vi "REWORK_add_values_to_operations.vi"(7 "REPORT_all_info":T1, 10 "operation_statuses":T3[](array[typedef]), 11 "operations":string[][](array[string])) -> (2 "record_statuses":T3[](array[typedef]), 3 "ItemNames":string[][](array[string]))   [LabVIEW 2019]
uses:
  REWORK_gear_statuses.ctl
  REWORK_all_info.ctl
  MAIN/REWORK_header_data_display.ctl
  REWORK_references.ctl
  <userlib>/_OpenG.lib/array/array.llb/Reverse 2D Array (String)__ogtk.vi
  <userlib>/_OpenG.lib/array/array.llb/Filter 1D Array with Scalar (String)__ogtk.vi
  _misc/AULocalize/SubVIs/Get Localized Phrase Compact Interface 1D.vi
  _misc/AULocalize/SubVIs/Get Localized Phrase Compact Interface 2D.vi
panel:
  # "GEAR INFO SUMMARY"
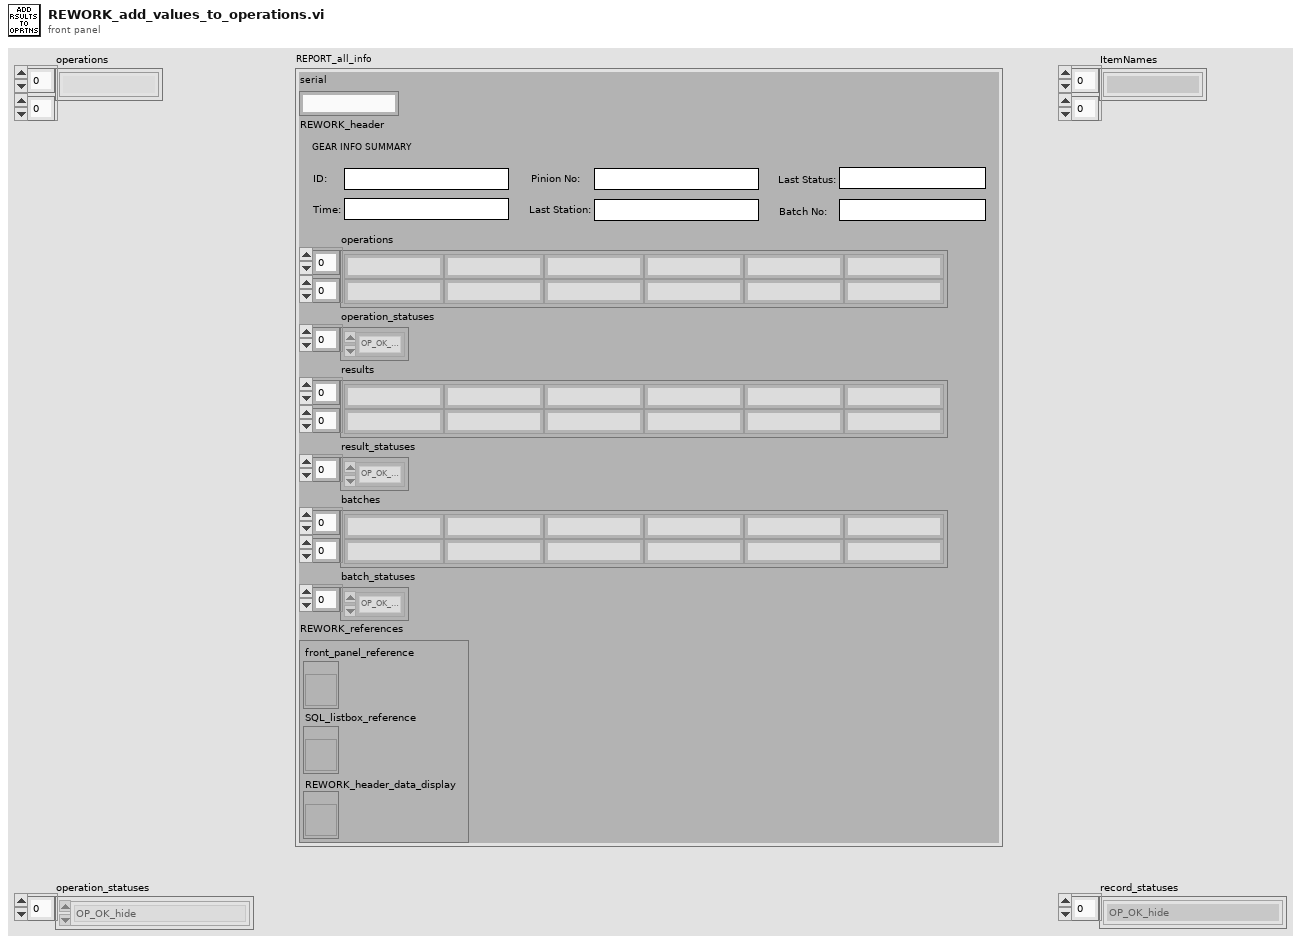
[diagram p1: front panel]
types:
  T1 = typedef "REWORK_all_info.ctl" = cluster{"serial":string, "REWORK_header":T2, "operations":string[][], "operation_statuses":T3[], "results":string[][], "result_statuses":T3[], "batches":string[][], "batch_statuses":T3[], "REWORK_references":T4}
  T2 = typedef "REWORK_header_data_display.ctl" = cluster{"ID":string, "creation_time":string, "last_station":string, "last_status":string, "pinion_serial":string, "batch_code":string}
  T3 = typedef "REWORK_gear_statuses.ctl" = enum16{"OP_OK_hide", "OP_OK_show", "OP_NOK_hide", "OP_NOK_show", "OP_interrupted_hide", "OP_interrupted_show", "OP_in_operation_hide", "OP_in_operation_show", "OP_unexpected_hide", "OP_unexpected_show", "RE_REAL_OK", "RE_REAL_NOK", "RE_STRING", "RE_sub_header", "RE_no_data", "RE_unexpected", "BA_sub_header", "BA_data", "BA_no_data"}
  T4 = typedef "REWORK_references.ctl" = cluster{"front_panel_reference":refnum<vi>, "SQL_listbox_reference":refnum<vi>, "REWORK_header_data_display":refnum<vi>}
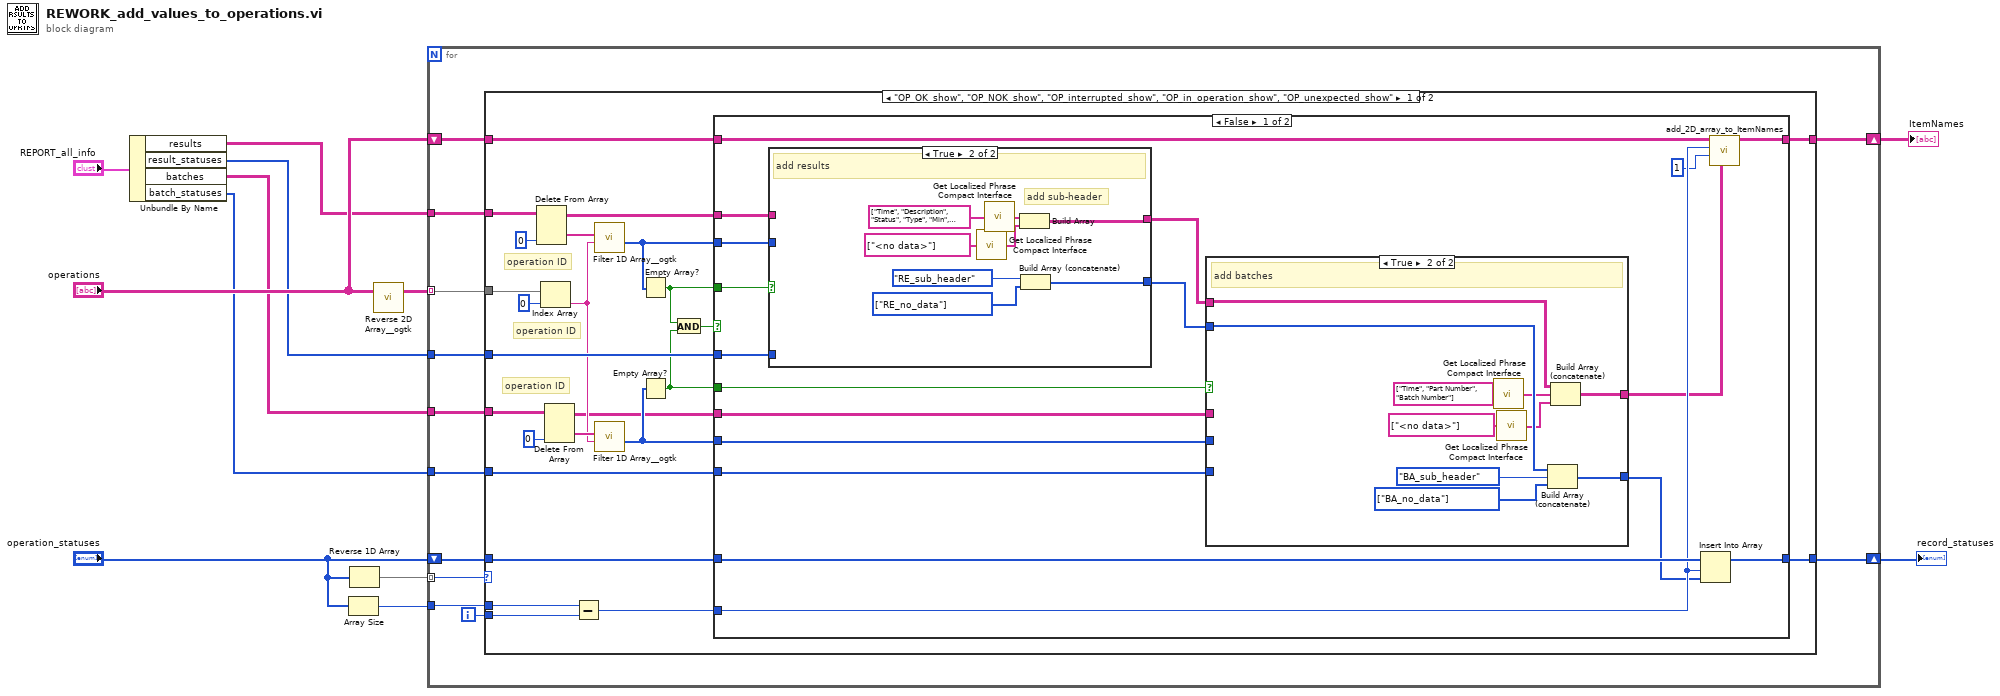
[diagram p0: block diagram]
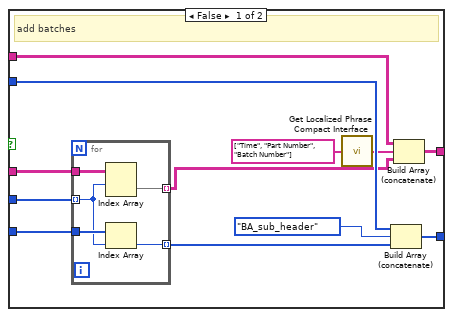
[diagram p2: hidden frame]
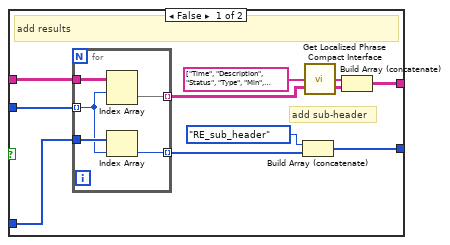
[diagram p3: hidden frame]
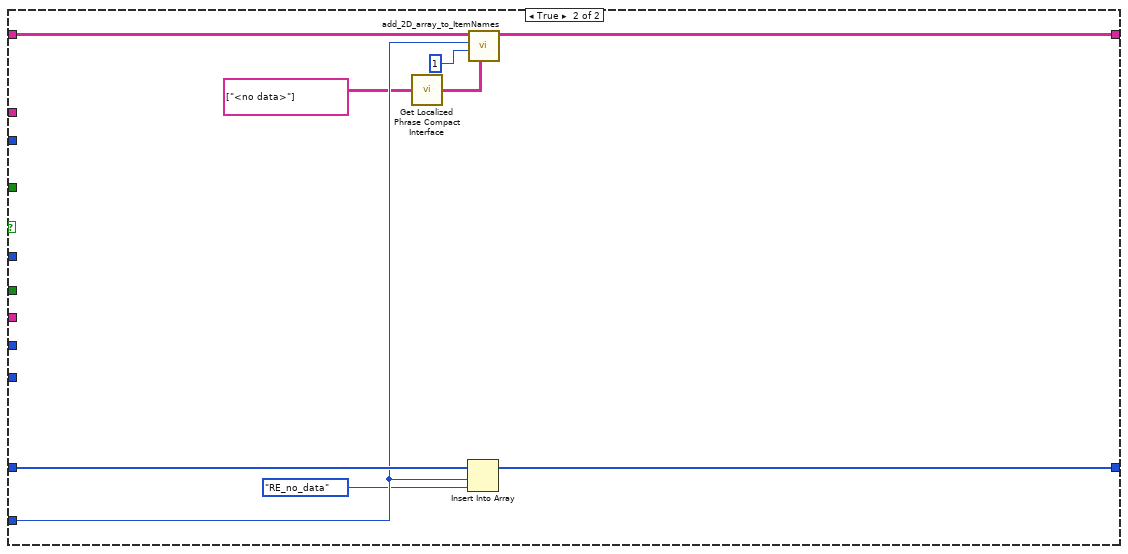
[diagram p4: hidden frame]
diagram:
  n1 = Unbundle By Name("REPORT_all_info") -> ("results"=w4:string[][], "result_statuses"=w3:T3[], "batches"=w2:string[][], "batch_statuses"=w1:T3[])
  n2 = Array Size(array="operation_statuses") -> (size(s)=w10:i32)
  n3 = Reverse 1D Array(array="operation_statuses") -> (reversed array=w12:T3[])
  n4 = call-poly <userlib>:"Reverse 2D Array__ogtk.vi"("Array"="operations") -> ("Reversed Array"=w7:string[][])  [unwired: 2 in]
  n5 = for {
    tunnel: w12 -> [w24] mode=indexing
    tunnel: w4 -> [w21]
    tunnel: w3 -> [w20]
    tunnel: w7 -> [w22] mode=indexing
    tunnel: w10 -> [w17]
    shift-right: [w16] -> w9
    shift-left: "operations" -> [w23]
    shift-right: [w15] -> w6
    shift-left: "operation_statuses" -> [w18]
    tunnel: w2 -> [w14]
    tunnel: w1 -> [w13]
    i -> [w19]
    n6 = case shown="\"OP_OK_show\", \"OP_NOK_show\", \"OP_interrupted_show\", \"OP_in_operation_show\", \"OP_unexpected_show\"" w24 {
      tunnel: w23 -> [w42 w128]
      tunnel: w22 -> [w49 _]
      tunnel: w21 -> [w38 _]
      tunnel: w20 -> [w47 _]
      tunnel: w19 -> [w45 _]
      tunnel: w18 -> [w44 w127]
      tunnel: w17 -> [w46 _]
      tunnel: [w41 w128] -> w16
      tunnel: [w43 w127] -> w15
      tunnel: w14 -> [w34 _]
      tunnel: w13 -> [w28 _]
      frame "OP_OK_show", "OP_NOK_show", "OP_interrupted_show", "OP_in_operation_show", "OP_unexpected_show" {
        # "operation ID"
        # "operation ID"
        # "operation ID"
        n7 = Delete From Array(array=w38, index (col)=0 ("disabled index (col)")) -> (deleted portion=w36:string[], array with subset deleted=w35:string[][])  [unwired: 2 in]
        n8 = Index Array(array=w49, index=0) -> (element=w31:string)
        n9 = Delete From Array(array=w34, index (col)=0 ("disabled index (col)")) -> (deleted portion=w32:string[], array with subset deleted=w25:string[][])  [unwired: 2 in]
        n10 = Subtract(x=w46, y=w45) -> (x-y=w40:i32)
        n11 = call-poly <userlib>:"Filter 1D Array__ogtk.vi"("items to filter"=w31, "array"=w36) -> ("filtered item indices"=w39:i32[])  [unwired: 4 in, 1 out]
        n12 = call-poly <userlib>:"Filter 1D Array__ogtk.vi"("items to filter"=w31, "array"=w32) -> ("filtered item indices"=w29:i32[])  [unwired: 4 in, 1 out]
        n13 = Empty Array?(array=w39) -> (empty?=w27:bool)
        n14 = Empty Array?(array=w29) -> (empty?=w26:bool)
        n15 = And(x=w27, y=w26) -> (x .and. y?=w30:bool)
        n16 = case shown="False" w30 {
          tunnel: w35 -> [w67 _]
          tunnel: w47 -> [w66 _]
          tunnel: w39 -> [w65 _]
          tunnel: w44 -> [w64 w126]
          tunnel: [w63 w125] -> w43
          tunnel: w42 -> [w62 w124]
          tunnel: [w61 w123] -> w41
          tunnel: w40 -> [w60 w122]
          tunnel: w29 -> [w51 _]
          tunnel: w28 -> [w50 _]
          tunnel: w27 -> [w58 _]
          tunnel: w26 -> [w57 _]
          tunnel: w25 -> [w52 _]
          frame False {
            n17 = case shown="True" w58 {
              tunnel: w67 -> [w104 _]
              tunnel: w66 -> [w103 _]
              tunnel: w65 -> [w102 _]
              tunnel: [w99 w115] -> w56
              tunnel: [w97 w112] -> w54
              frame False {
                # "add sub-header"
                # "add results"
                n18 = for {
                  tunnel: w104 -> [w109]
                  tunnel: w103 -> [w108]
                  tunnel: w102 -> [w107] mode=indexing
                  tunnel: [w106] -> w101 mode=indexing
                  tunnel: [w105] -> w98 mode=indexing
                  n19 = Index Array(array=w109, index (row)=w107) -> (element=w106:string[])  [unwired: 1 in]
                  n20 = Index Array(array=w108, index=w107) -> (element=w105:T3)
                }
                n21 = Build Array (concatenate)(REWORK_gear_statuses."RE_sub_header" ("REPORT_GEAR_statuses"), w98) -> (w97:T3[])
                n22 = call-poly "Get Localized Phrase Compact Interface.vi"("Key"=string[] ["Time", "Description", "Status", "Type", "Min", "Value", "Max", "Unit"]) -> ("Translated Phrase"=w95:string[])
                n23 = Build Array (concatenate)(w95, w101) -> (w99:string[][])
              }
              frame True {
                w113 = T3[] [enum."RE_no_data"] items=["OP_OK_hide", "OP_OK_show", "OP_NOK_hide", "OP_NOK_show", "OP_interrupted_hide", "OP_interrupted_show", "OP_in_operation_hide", "OP_in_operation_show", "OP_unexpected_hide", "OP_unexpected_show", "RE_REAL_OK", "RE_REAL_NOK", "RE_STRING", "RE_sub_header", "RE_no_data", "RE_unexpected", "BA_sub_header", "BA_data", "BA_no_data"] ("Array")
                # "add sub-header"
                # "add results"
                n24 = call-poly "Get Localized Phrase Compact Interface.vi"("Key"=string[] ["<no data>"] ("element")) -> ("Translated Phrase"=w110:string[])
                n25 = call-poly "Get Localized Phrase Compact Interface.vi"("Key"=string[] ["Time", "Description", "Status", "Type", "Min", "Value", "Max", "Unit"]) -> ("Translated Phrase"=w111:string[])
                n26 = Build Array(w111, w110) -> (w115:string[][])
                n27 = Build Array (concatenate)(REWORK_gear_statuses."RE_sub_header" ("REPORT_GEAR_statuses"), w113) -> (w112:T3[])
              }
            }
            n28 = case shown="True" w57 {
              tunnel: w56 -> [w75 w92]
              tunnel: [w76 w90] -> w55
              tunnel: w54 -> [w74 w91]
              tunnel: [w77 w89] -> w53
              tunnel: w52 -> [w72 _]
              tunnel: w51 -> [w71 _]
              tunnel: w50 -> [w70 _]
              frame False {
                # "add batches"
                n29 = for {
                  tunnel: w72 -> [w84]
                  tunnel: w70 -> [w83]
                  tunnel: w71 -> [w82] mode=indexing
                  tunnel: [w81] -> w73 mode=indexing
                  tunnel: [w80] -> w69 mode=indexing
                  n30 = Index Array(array=w84, index (row)=w82) -> (element=w81:string[])  [unwired: 1 in]
                  n31 = Index Array(array=w83, index=w82) -> (element=w80:T3)
                }
                n32 = call-poly "Get Localized Phrase Compact Interface.vi"("Key"=string[] ["Time", "Part Number", "Batch Number"]) -> ("Translated Phrase"=w68:string[])
                n33 = Build Array (concatenate)(w74, REWORK_gear_statuses."BA_sub_header" ("REPORT_GEAR_statuses"), w69) -> (w77:T3[])
                n34 = Build Array (concatenate)(w75, w68, w73) -> (w76:string[][])
              }
              frame True {
                w88 = T3[] [enum."BA_no_data"] items=["OP_OK_hide", "OP_OK_show", "OP_NOK_hide", "OP_NOK_show", "OP_interrupted_hide", "OP_interrupted_show", "OP_in_operation_hide", "OP_in_operation_show", "OP_unexpected_hide", "OP_unexpected_show", "RE_REAL_OK", "RE_REAL_NOK", "RE_STRING", "RE_sub_header", "RE_no_data", "RE_unexpected", "BA_sub_header", "BA_data", "BA_no_data"] ("Array")
                # "add batches"
                n35 = call-poly "Get Localized Phrase Compact Interface.vi"("Key"=string[] ["Time", "Part Number", "Batch Number"]) -> ("Translated Phrase"=w86:string[])
                n36 = call-poly "Get Localized Phrase Compact Interface.vi"("Key"=string[] ["<no data>"] ("element")) -> ("Translated Phrase"=w85:string[])
                n37 = Build Array (concatenate)(w91, REWORK_gear_statuses."BA_sub_header" ("REPORT_GEAR_statuses"), w88) -> (w89:T3[])
                n38 = Build Array (concatenate)(w92, w86, w85) -> (w90:string[][])
              }
            }
            n39 = Insert Into Array(array=w64, index=w60, new element=w53) -> (w63:T3[])
            n40 = call "add_2D_array_to_ItemNames.vi"("2D_array"=w55, "column"=1, "row"=w60, "ItemNames_in"=w62) -> ("ItemNames_out"=w61:string[][])  [unwired: 7 in]
          }
          frame True {
            n41 = call-poly "Get Localized Phrase Compact Interface.vi"("Key"=string[][] [["<no data>"]] ("2D_array")) -> ("Translated Phrase"=w118:string[][])
            n42 = Insert Into Array(array=w126, index=w122, new element=REWORK_gear_statuses."RE_no_data" ("new element/subarray")) -> (w125:T3[])
            n43 = call "add_2D_array_to_ItemNames.vi"("2D_array"=w118, "column"=1, "row"=w122, "ItemNames_in"=w124) -> ("ItemNames_out"=w123:string[][])  [unwired: 7 in]
          }
        }
      }
      frame Default {
      }
    }
  }
  "ItemNames" <- w9
  "record_statuses" <- w6
